vi "Target VI Read.vi"(4 "error in (no error)":errorcluster, 6 "Container State":T2, 7 "Display State In":T1) -> (0 "error out":errorcluster, 2 "Value":path, 3 "Display State Out":T1)   [LabVIEW 2009, in "Jump Button (System).xctl"]
uses:
  <vilib>/Navigation Controls/Jump Button System/Jump Button (System).xctl
  <vilib>/_xctls/Container State.ctl
  <vilib>/Navigation Controls/Jump Button System/Jump Button State.ctl
  <vilib>/Navigation Controls/NI_Navigation.lvlib
  <vilib>/_xctls/XControlSupport.lvlib
panel:
  # "Replace the Value Indicator below with an Indicator of desired type.\nDo not remove this Indicator or the others from the connector pane. \nDo not change the connector pane pattern.\nThe Value Indicator should always be the second terminal from top on the output side in the connector pane."
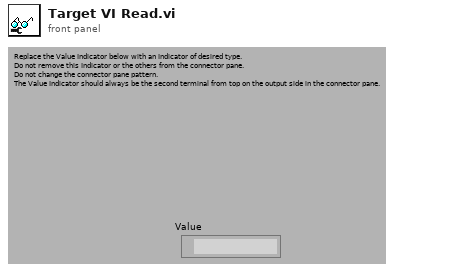
[diagram p1: front panel]
types:
  T1 = typedef "Jump Button (System).xctl/Jump Button State.ctl" = cluster{"Button Text":string, "Absolute Path":path, "Relative Path":path}
  T2 = typedef "XControlSupport.lvlib/Container State.ctl" = cluster{"Indicator?":bool, "Run Mode?":bool, " Refnum":refnum<vi>}
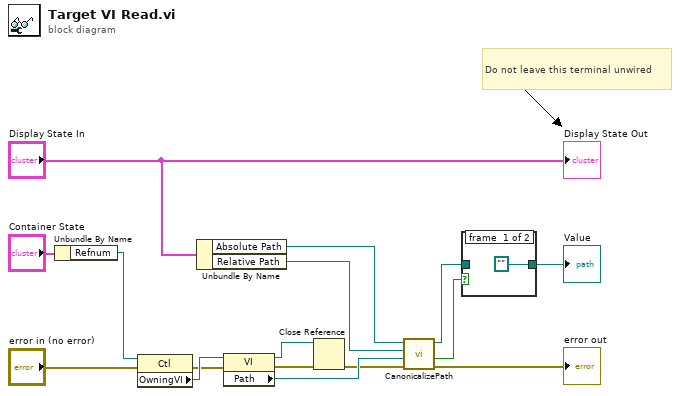
[diagram p0: block diagram]
diagram:
  # "Do not leave this terminal unwired"
  n1 = Unbundle By Name("Container State") -> ("Refnum"=w16:refnum<vi>)
  n2 = property class="Ctl"(reference=w16, error in="error in (no error)") -> (error out=w14:errorcluster, "OwningVI"=w15:refnum<vi>)  [unwired: 1 out]
  n3 = Unbundle By Name("Display State In") -> ("Absolute Path"=w12:path, "Relative Path"=w11:path)
  n4 = property class="VI"(reference=w15, error in=w14) -> (reference out=w8:refnum<vi>, error out=w13:errorcluster, "Path"=w10:path)
  n5 = Close Reference(reference=w8, error in (no error)=w13) -> (error out=w9:errorcluster)
  n6 = call <vilib>:"CanonicalizePath.vi"("error in (no error)"=w9, "VI Path"=w10, "Relative Path"=w11, "Absolute Path"=w12) -> ("error out"=→"error out":errorcluster, "Found?"=w7:bool, "Canonicalized Path Out"=w6:path)  [unwired: 5 in]
  n7 = case shown="False" w7 {
    tunnel: w6 -> [_ w18]
    tunnel: [path "" w18] -> w2
    frame #0 {
    }
    frame #1 {
    }
  }
  "Value" <- w2
  "Display State Out" <- "Display State In"
